vi "Test_Draw_Ellipse_ARGB.vi"(8 "error in (no error)":errorcluster, 11 "Test Case In":refnum<class "Image.lvclass">) -> (0 "error out":errorcluster, 3 "Test Case Out":refnum<class "Image.lvclass">)   [LabVIEW 2020, in "g_ar_toolkit.test.lvlib" / "Image.lvclass"]
uses:
  Image.lvclass
  Image.lvclass/Image.ctl
  g_ar_toolkit.image/g_ar_toolkit.image.lvlib
  g_ar_toolkit.image/CreateEmptyImageARGB.vi
  g_ar_toolkit.image/ARGB Colour.ctl
  g_ar_toolkit.image/Image Size (Fixed).ctl
  g_ar_toolkit.image/Line Type.ctl
  g_ar_toolkit.image/Image Point (Fixed).ctl
  g_ar_toolkit.image/Ellipse Angles.ctl
  4993e8ee-a06a-463a-9684-69129f64d5ce.vi
panel:
  out "Picture":picture
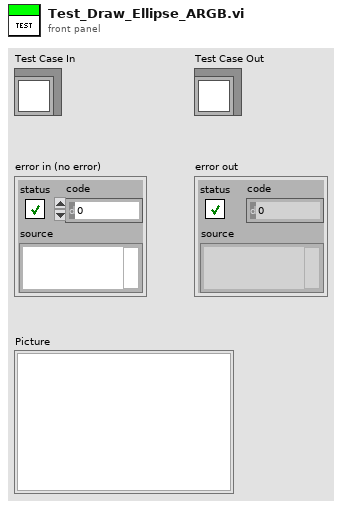
[diagram p1: front panel]
types:
  T1 = typedef "g_ar_toolkit.image.lvlib/Ellipse Angles.ctl" = cluster{"Rotation":dbl, "Start":dbl, "Stop":dbl}
  T2 = typedef "g_ar_toolkit.image.lvlib/Image Size (Fixed).ctl" = cluster{"Width":u16, "Height":u16}
  T3 = typedef "g_ar_toolkit.image.lvlib/Image Point (Fixed).ctl" = cluster{"x":i32, "y":i32}
  T4 = typedef "g_ar_toolkit.image.lvlib/Line Type.ctl" = enum8{"FILLED", "LINE_4", "LINE_8", "LINE_AA"}
  T5 = typedef "g_ar_toolkit.image.lvlib/ARGB Colour.ctl" = cluster{"Alpha":u8, "RGB":u32}
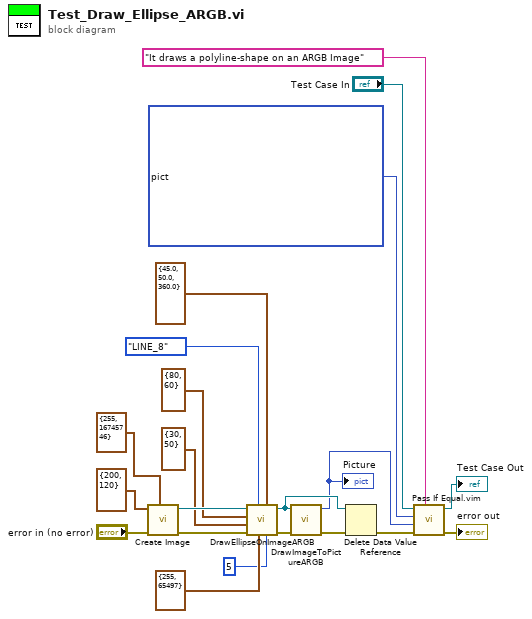
[diagram p0: block diagram]
diagram:
  n1 = call-poly "Create Image.vi"("Colour (Default: Black)"=T5 {"Alpha"=255, "RGB"=16745746}, "error in (no error)"="error in (no error)", "Preallocated Image Size (Default: 0,0)"=T2 {"Width"=200, "Height"=120}) -> ("error out"=w14:errorcluster, "New ARGB Image"=w15:refnum<data-value>)  [unwired: 7 in]
  n2 = call "DrawEllipseOnImageARGB.vi"("Thickness (Default: 1)"=u16 5, "Ellipse Angles (Default: No rotation & full)"=T1 {"Rotation"=45.0, "Start"=50.0, "Stop"=360.0}, "ARGB Colour"=T5 {"Alpha"=255, "RGB"=65497}, "OpenCV Line Type (Default LINE_8)"=Line_Type."LINE_8", "error in (no error)"=w14, "Axes"=T2 {"Width"=30, "Height"=50}, "Centre"=T3 {"x"=80, "y"=60}, "ARGB Image"=w15) -> ("error out"=w12:errorcluster, "ARGB Image (Duplicate)"=w13:refnum<data-value>)  [unwired: 2 in]
  n3 = call "DrawImageToPictureARGB.vi"("error in (no error)"=w12, "ARGB Image Source"=w13) -> ("error out"=w11:errorcluster, "Picture"=w6:picture)  [unwired: 8 in]
  "Picture" <- w6
  n4 = Delete Data Value Reference(data value reference=w13, error in=w11) -> (error out=w17:errorcluster)  [unwired: 1 out]
  n5 = call "Pass If Equal.vim"("Description"="It draws a polyline-shape on an ARGB Image", "error in (no error)"=w17, "Actual"=w6, "Expected"=picture bytes[72030] ("Picture"), "LUnit Test Case In"="Test Case In") -> ("error out"=→"error out":errorcluster, "LUnit Test Case Out"=→"Test Case Out":refnum<class "Image.lvclass">)  [unwired: 5 in]
